vi "SRS Lockin.vi"(1 "Action":T4=enum."Identify", 2 "Parameters":variant) -> (6 "Output":variant, 7 "Stop":bool)   [LabVIEW 2020]
uses:
  Sub Controls/Instrument Actions.ctl
  Sub Controls/Public.ctl
  Sub Controls/Instrument Match.ctl
  SubVIs/Lockin Channels.ctl
  Sub Controls/Scan Output.ctl
  Sub Controls/Instrument IDN.ctl
  Sub Controls/User Event Command.ctl
panel:
  in  "Factory Reset":bool
  out "Channel Index":i32
  in  "Channels":T1={"X"=TRUE, "X&Y"=FALSE, "R"=FALSE, "R & ϴ"=FALSE}
  out "Title":string="Stanford Research Lockin"
  in  "VISA resource name":refnum<visa-resource-name>
  in  "Instruments":T2[](array[typedef])=[{"Model"="SR8[35]0", "Manufacturer"="Stanford_Research_Systems", "Term Character"="", "Wait Time (mS)"=0, "Wait for SRQ"=FALSE, "Type"="Lockin"}, {"Model"="SR844", "Manufacturer"="Stanford_Research_Systems", "Term Character"="", "Wait Time (mS)"=0, "Wait for SRQ"=FALSE, "Type"="Lockin"}, {"Model"="SR865A*", "Manufacturer"="Stanford_Research_Systems", "Term Character"="", "Wait Time (mS)"=0, "Wait for SRQ"=FALSE, "Type"="Lockin"}, {"Model"="SR860", "Manufacturer"="Stanford_Research_Systems", "Term Character"="", "Wait Time (mS)"=0, "Wait for SRQ"=FALSE, "Type"="Lockin"}]
  out "Model":string
  in  "Address":u16(ring)
  in  "Public":T3
  out "Measurement":dbl[](array[numeric]) format="%^.3e"
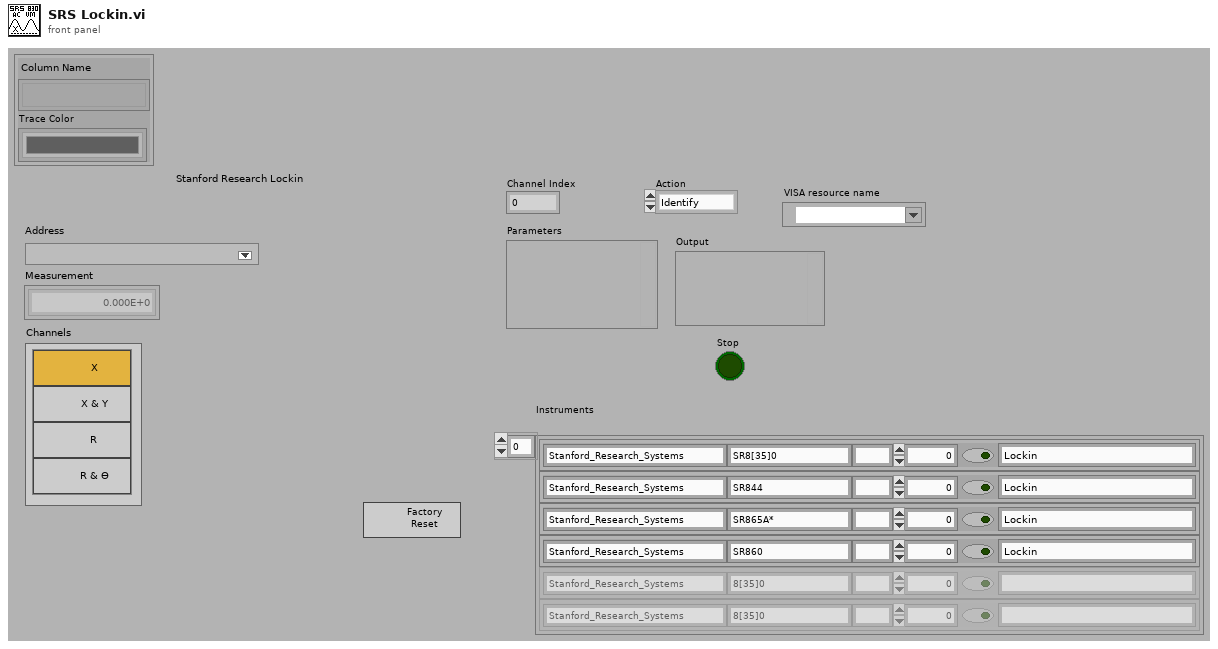
[diagram p1: front panel]
types:
  T1 = typedef "Lockin Channels.ctl" = cluster{"X":bool, "X&Y":bool, "R":bool, "R & ϴ":bool}
  T2 = typedef "Instrument Match.ctl" = cluster{"Model":string, "Manufacturer":string, "Term Character":string, "Wait Time (mS)":u32, "Wait for SRQ":bool, "Type":string}
  T3 = typedef "Public.ctl" = cluster{"Column Name":string[], "Trace Color":u32[]}
  T4 = typedef "Instrument Actions.ctl" = enum16{"Scan", "Identify", "New", "Configure", "Initialize", "Test", "Read", "Close"}
  T5 = typedef "Scan Output.ctl" = cluster{"Manufacturer":string, "Model":string, "Info":string, "Revision":string, "error out":errorcluster}
  T6 = typedef "Instrument IDN.ctl" = cluster{"VISA Address":string, "Status":u16, "Manufacturer":string, "Model":string, "Info":string, "Info 2":string, "Misc Data":variant}
  T7 = typedef "User Event Command.ctl" = enum32{"Stop Config"}
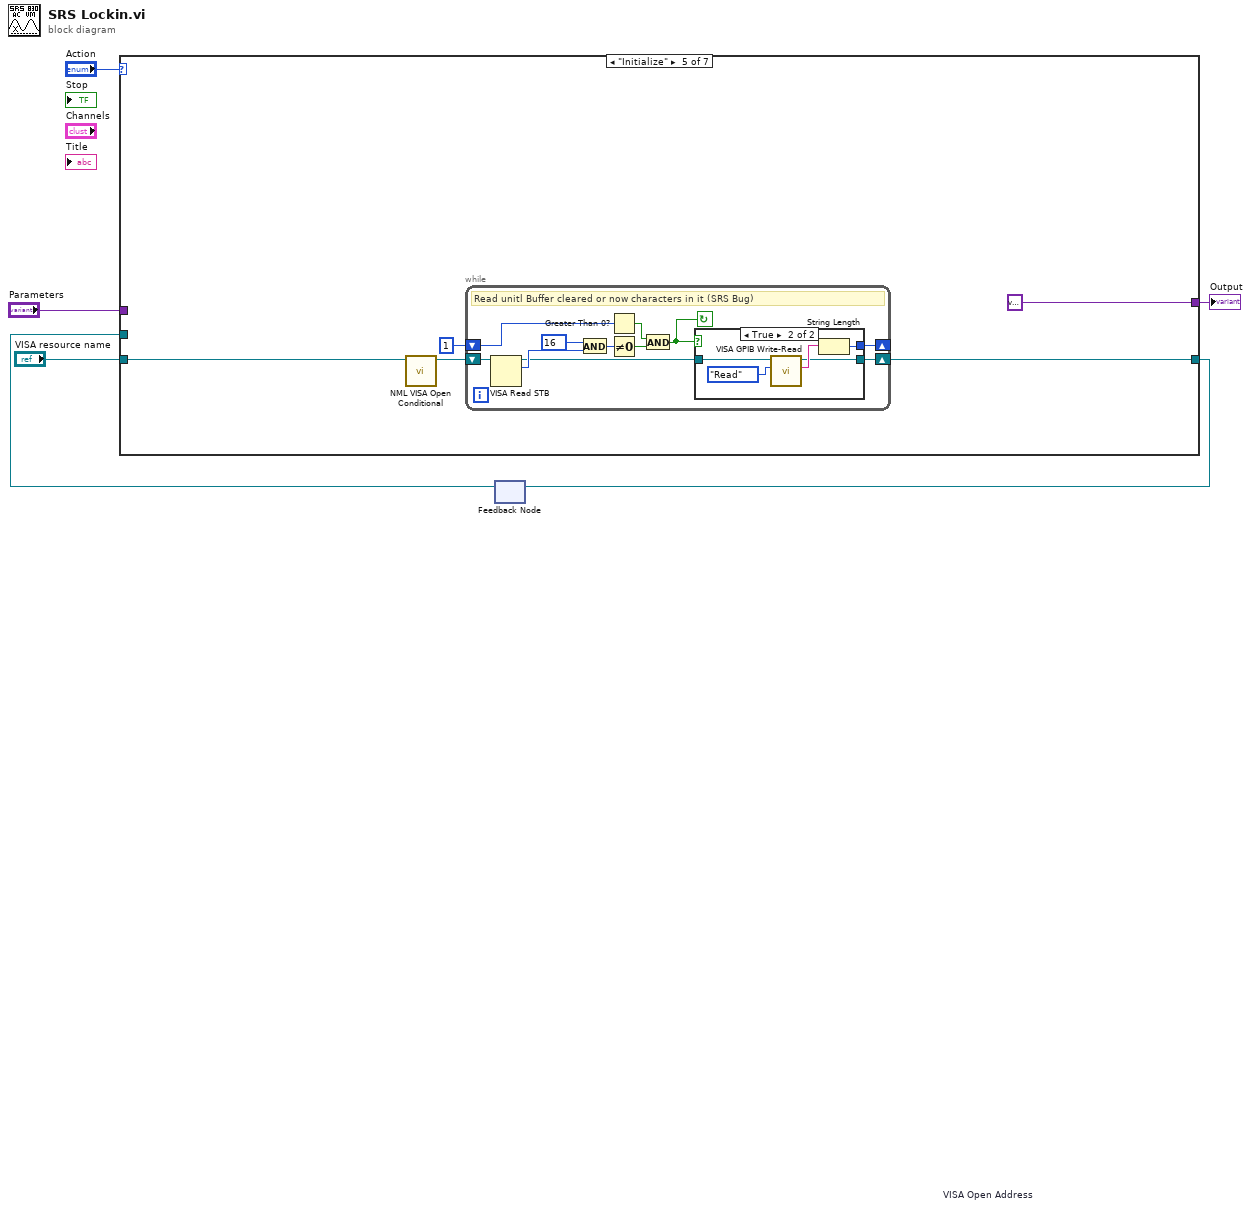
[diagram p0: block diagram]
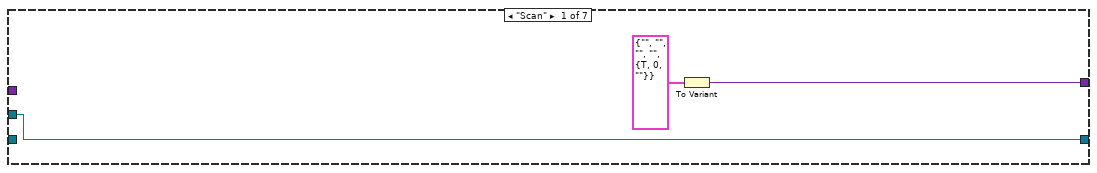
[diagram p2: hidden frame]
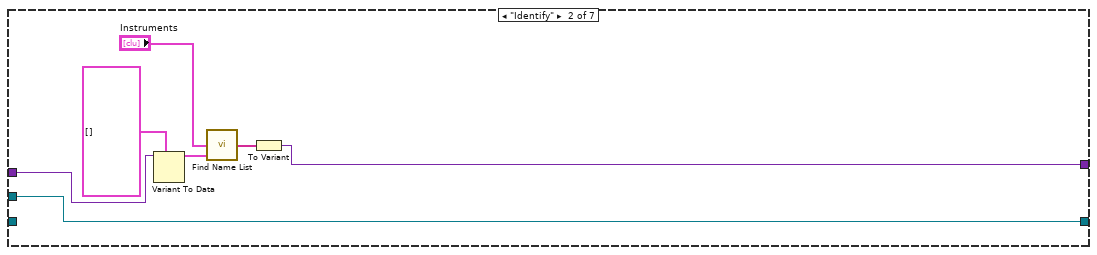
[diagram p3: hidden frame]
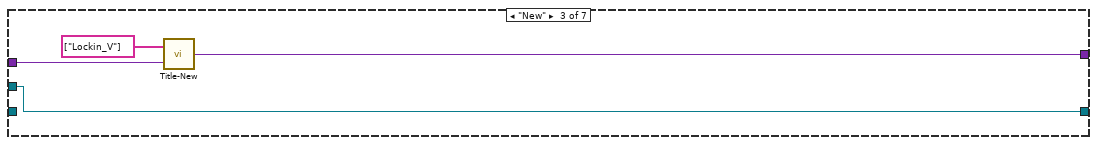
[diagram p4: hidden frame]
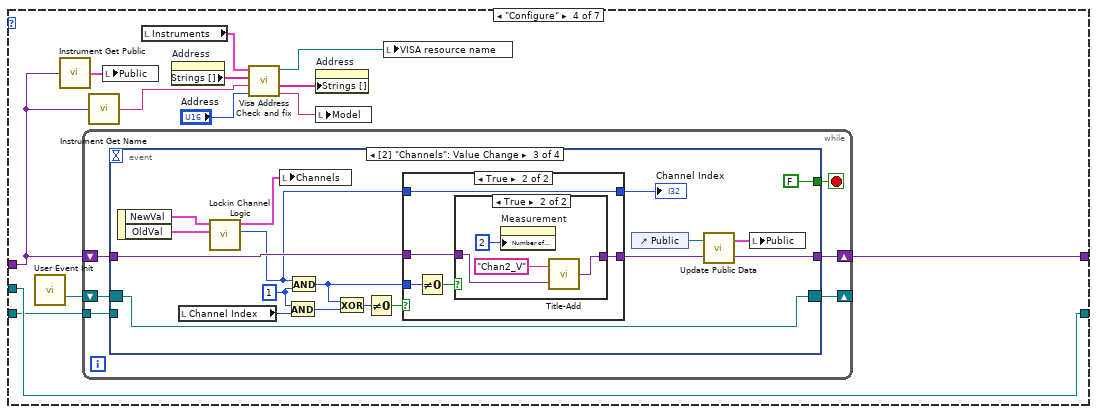
[diagram p5: hidden frame]
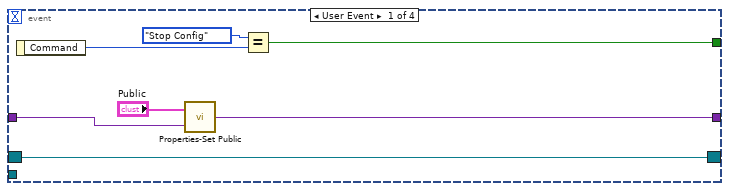
[diagram p6: hidden frame]
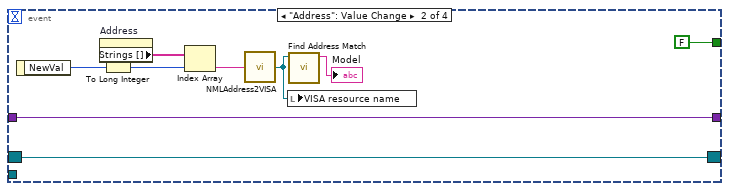
[diagram p7: hidden frame]
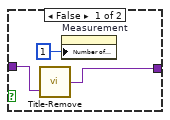
[diagram p9: hidden frame]
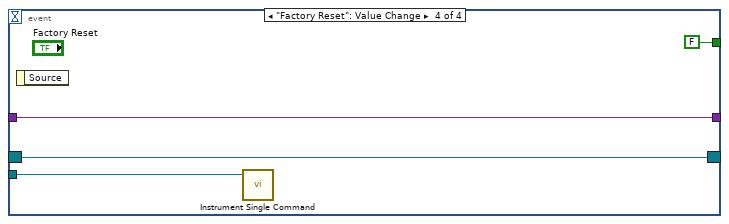
[diagram p10: hidden frame]
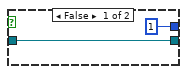
[diagram p11: hidden frame]
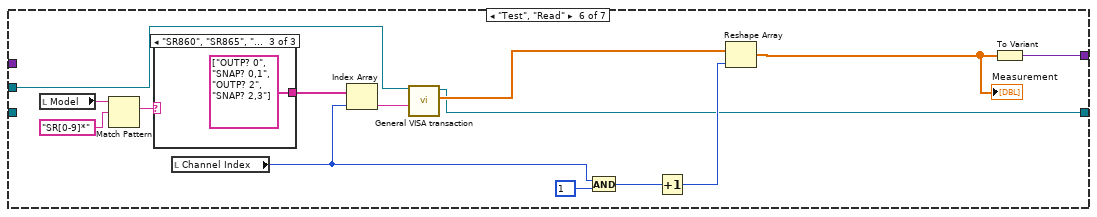
[diagram p12: hidden frame]
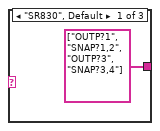
[diagram p13: hidden frame]
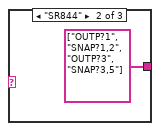
[diagram p14: hidden frame]
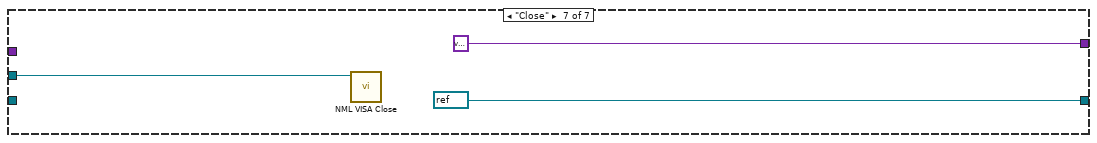
[diagram p15: hidden frame]
diagram:
  n1 = feedback #1 "VISA Open Address"() -> (w2:refnum<visa-resource-name>)  [unwired: 1 in]
  n2 = case shown="\"Initialize\"" "Action" {
    tunnel: [w8 w16 w19 w22 w92 w115 refnum<visa-resource-name> refnum ("Open VISA Resource name")] -> w3
    tunnel: w2 -> [w8 w16 w19 w22 _ w116 w132]
    tunnel: "Parameters" -> [_ w13 w20 w26 _ _ _]
    tunnel: [w7 w15 w17 w33 variant ("Variant") w128 variant ("Variant")] -> w5
    tunnel: "VISA resource name" -> [_ _ _ w21 w95 _ _]
    frame "Scan" {
      n3 = To Variant(anything=T5 {"Manufacturer"="", "Model"="", "Info"="", "Revision"="", "error out"={"status"=TRUE, "code"=0, "source"=""}} ("Scan Output")) -> (Variant=w7:variant)
    }
    frame "Identify" {
      n4 = Variant To Data(type=T6[] [], Variant=w13) -> (data=w11:T6[])  [unwired: 1 in, 1 out]
      n5 = call "Find Name List.vi"("Bus Scan"=w11, "Instruments"="Instruments") -> ("Names"=w10:string[])  [unwired: 1 in]
      n6 = To Variant(anything=w10) -> (Variant=w15:variant)
    }
    frame "New" {
      n7 = call "Title-New.vi"("Parameters"=w20, "Array"=string[] ["Lockin_V"]) -> ("Instrument Prop"=w17:variant)
    }
    frame "Configure" {
      n8 = call "User Event Init.vi"() -> ("Event Registration Refnum"=w31:refnum<event-registration>)  [unwired: 14 in, 1 out]
      n9 = call "Instrument Get Public.vi"("Variant"=w26) -> ("Public"=w32:T3)
      n10 = while {
        shift-right: [w39] -> w33
        shift-left: w26 -> [w38]
        shift-right: [w35] -> _
        shift-left: w31 -> [w36]
        tunnel: w21 -> [w34]
        stop <- w37 stop-if-true
        n11 = event shown="[2] \"Channels\": Value Change" {
          selector: w36 -> [w40 w55 w72 w89]
          dyn-events: [w40 w55 w72 w89] -> w35
          timeout: _ -> [_ _ _ _]
          tunnel: [w42 FALSE FALSE FALSE] -> w37
          tunnel: w38 -> [w45 w49 w73 w90]
          tunnel: [w46 w49 w70 w90] -> w39
          tunnel: w34 -> [_ _ _ w88]
          event User Event {
            n12 = event-data() -> ("Command"=w44:T7)  [unwired: 1 in]
            n13 = call "Properties-Set Public.vi"("Variant"=w45, "New Public"="Public") -> ("Variant 2"=w46:variant)
            n14 = Equal?(x=User_Event_Command."Stop Config", y=w44) -> (x = y?=w42:bool)
          }
          event "Address": Value Change {
            n15 = event-data() -> ("NewVal"=w53:u16)  [unwired: 1 in]
            n16 = property on="Address" class="Ring (strict)"() -> ("Strings []"=w52:string[])  [unwired: 2 in, 2 out]
            n17 = To Long Integer(number=w53) -> (32bit integer=w47:i32)
            n18 = Index Array(array=w52, index=w47) -> (element=w51:string)
            n19 = call "NMLAddress2VISA.vi"("NML Address"=w51) -> ("VISA resource name"=w48:refnum<visa-resource-name>)
            n20 = local write "VISA resource name"(w48) -> ()
            n21 = call "Find Address Match.vi"("VISA resource name"=w48) -> ("Model"=→"Model":string)  [unwired: 3 in, 3 out]
          }
          event Value Change {
            w62 = 1 ("y")
            n22 = event-data() -> ("NewVal"=w66:T1, "OldVal"=w65:T1)  [unwired: 1 in]
            n23 = local read "Channel Index"() -> (w63:i32)
            n24 = call "Lockin Channel Logic.vi"("Old Channels"=w65, "New Channels"=w66) -> ("index of element"=w57:i32, "Channels Out"=w64:T1)  [unwired: 8 in]
            n25 = local write "Channels"(w64) -> ()
            n26 = And(x=w62, y=w63) -> (x .and. y?=w61:i32)
            n27 = And(x=w57, y=w62) -> (x .and. y?=w58:i32)
            n28 = Exclusive Or(1:w61, 2:w58) -> (0:w59:i32)
            n29 = Not Equal To 0?(x=w59) -> (x != 0?=w60:bool)
            n30 = case shown="True" w60 {
              tunnel: w73 -> [w74 w80]
              tunnel: [w74 w79] -> w71
              tunnel: w58 -> [_ w77]
              tunnel: [w75 w76] -> w56
              tunnel: w57 -> [w75 w76]
              frame False {
              }
              frame True {
                n31 = Not Equal To 0?(x=w77) -> (x != 0?=w78:bool)
                n32 = case shown="True" w78 {
                  tunnel: w80 -> [w83 w87]
                  tunnel: [w82 w86] -> w79
                  frame False {
                    n33 = call "Title-Remove.vi"("Parameters"=w83) -> ("Variant"=w82:variant)  [unwired: 1 in]
                    n34 = property on="Measurement" class="Arr (strict)"("Number of Columns"=u32 1) -> ()  [unwired: 2 in, 2 out]
                  }
                  frame True {
                    n35 = property on="Measurement" class="Arr (strict)"("Number of Columns"=u32 2) -> ()  [unwired: 2 in, 2 out]
                    n36 = call "Title-Add.vi"("Parameters"=w87, "String"="Chan2_V") -> ("Variant"=w86:variant)
                  }
                }
              }
            }
            "Channel Index" <- w56
            n37 = control-ref of="Public"() -> (w68:refnum<vi>)
            n38 = call "Update Public Data.vi"("Variant In"=w71, "Public 2"=w68) -> ("Variant Out"=w70:variant, "Public"=w69:T3)
            n39 = local write "Public"(w69) -> ()
          }
          event "Factory Reset": Value Change {
            n40 = event-data() -> ()  [unwired: 1 in, 1 out]
            n41 = call "Instrument Single Command.vi"("VISA Name"=w88) -> ()  [unwired: 10 in, 1 out]
          }
        }
      }
      n42 = call "Instrument Get Name.vi"("Parameters"=w26) -> ("Type"=w27:string)
      n43 = local write "Public"(w32) -> ()
      n44 = local read "Instruments"() -> (w25:T2[])
      n45 = property on="Address" class="Ring (strict)"() -> ("Strings []"=w29:string[])  [unwired: 2 in, 2 out]
      n46 = call "Visa Address Check and fix.vi"("Address"="Address", "Name"=w27, "NML Addresses"=w29, "Instruments"=w25) -> ("Model"=w23:string, "NML Addresses"=w24:string[], "VISA resource name"=w28:refnum<visa-resource-name>)  [unwired: 3 out]
      n47 = property on="Address" class="Ring (strict)"("Strings []"=w24) -> ()  [unwired: 2 in, 2 out]
      n48 = local write "Model"(w23) -> ()
      n49 = local write "VISA resource name"(w28) -> ()
    }
    frame "Initialize" {
      n50 = call "NML VISA Open Conditional.vi"("VISA resource name"=w95) -> ("dup VISA Session"=w93:refnum<visa-resource-name>)  [unwired: 8 in, 2 out]
      n51 = while {
        shift-right: [w102] -> w92
        shift-left: w93 -> [w101]
        shift-right: [w99] -> _
        shift-left: 1 -> [w100]
        stop <- w98 continue-if-true
        # "Read unitl Buffer cleared or now characters in it (SRS Bug)"
        n52 = VISA Read STB(11:w101) -> (2:w106:u16, 3:w105:refnum<visa-resource-name>)  [unwired: 1 in, 1 out]
        n53 = And(x=u16 16, y=w106) -> (x .and. y?=w97:u16)
        n54 = Greater Than 0?(x=w100) -> (x > 0?=w103:bool)
        n55 = Not Equal To 0?(x=w97) -> (x != 0?=w107:bool)
        n56 = And(x=w103, y=w107) -> (x .and. y?=w98:bool)
        n57 = case shown="True" w98 {
          tunnel: w105 -> [w108 w111]
          tunnel: [1 w114] -> w99
          tunnel: [w108 w110] -> w102
          frame False {
          }
          frame True {
            n58 = call "VISA GPIB Write-Read.vi"("Action"=enum16{"Write", "Read", "Write & Read"}."Read", "VISA resource name"=w111) -> ("String Returned"=w113:string, "dup VISA Session"=w110:refnum<visa-resource-name>)  [unwired: 6 in, 2 out]
            n59 = String Length(string=w113) -> (length=w114:i32)
          }
        }
      }
    }
    frame "Test", "Read" {
      n60 = local read "Model"() -> (w124:string)
      n61 = Match Pattern(string=w124, regular expression="SR[0-9]*") -> (match substring=w125:string)  [unwired: 1 in, 3 out]
      n62 = case shown="\"SR860\", \"SR865\", \"SR865A\"" w125 {
        tunnel: [string[] ["OUTP?1", "SNAP?1,2", "OUTP?3", "SNAP?3,4"] ("array") string[] ["OUTP?1", "SNAP?1,2", "OUTP?3", "SNAP?3,5"] ("array") string[] ["OUTP? 0", "SNAP? 0,1", "OUTP? 2", "SNAP? 2,3"] ("array")] -> w123
        frame "SR830", Default {
        }
        frame "SR844" {
        }
        frame "SR860", "SR865", "SR865A" {
        }
      }
      n63 = local read "Channel Index"() -> (w117:i32)
      n64 = Index Array(array=w123, index=w117) -> (element=w122:string)
      n65 = call "General VISA transaction.vi"("Command String"=w122, "VISA Session"=w116) -> ("Measurement"=w127:dbl[], "dup VISA Session"=w115:refnum<visa-resource-name>)  [unwired: 4 in, 4 out]
      n66 = And(x=w117, y=1) -> (x .and. y?=w119:i32)
      n67 = Increment(x=w119) -> (x+1=w118:i32)
      n68 = Reshape Array(w127, w118) -> (w121:dbl[])
      "Measurement" <- w121
      n69 = To Variant(anything=w121) -> (Variant=w128:variant)
    }
    frame "Close" {
      n70 = call "NML VISA Close.vi"("VISA resource name"=w132) -> ()  [unwired: 10 in, 1 out]
    }
  }
  "Output" <- w5
  n71 = feedback-in #1(w3) -> ()
